vi "UpdateData.vi"(8 "error in (no error)":errorcluster, 10 "Select Conditions Criteria":T1, 11 "object in":refnum<class "TableLogger_Actor.lvclass">) -> (0 "error out":errorcluster, 2 "Data Clusters":variant[](array[variant]), 3 "object out":refnum<class "TableLogger_Actor.lvclass">)   [LabVIEW 2014, in "TableLogger_Actor.lvlib" / "TableLogger_Actor.lvclass"]
uses:
  TableLogger_Actor.lvclass
  SelectConditionCriteria.ctl
  TableLogger_SQLite_Actor/SelectConditions.ctl
  TableLogger_Actor.lvlib
panel:
  # "Connector Pane"
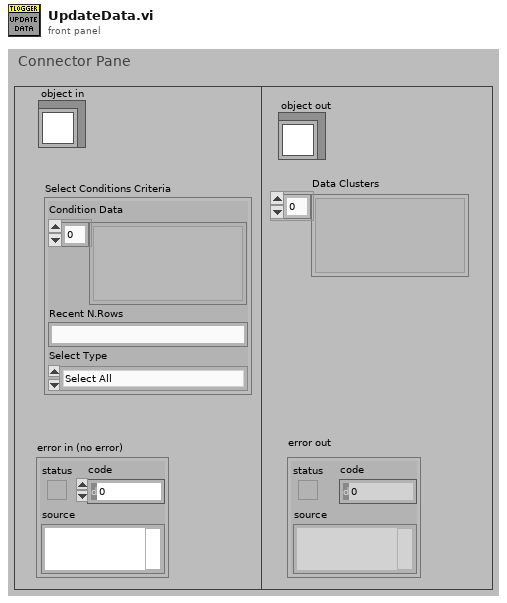
[diagram p1: front panel]
types:
  T1 = typedef "TableLogger_Actor.lvlib/SelectConditionCriteria.ctl" = cluster{"Condition Data":variant[], "Recent N.Rows":string, "Select Type":T2}
  T2 = typedef "TableLogger_Actor.lvlib/SelectConditions.ctl" = enum16{"Select All", "Select with AND Operator", "Select Most Recent Rows", "Select with OR Operator", "Select with BETWEEN Operator"}
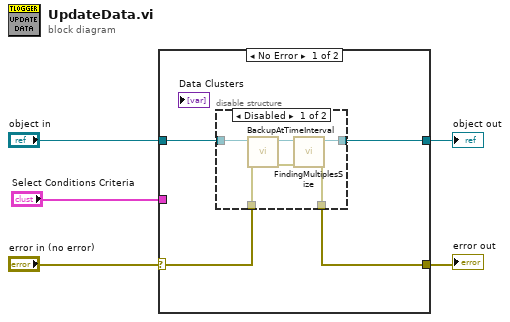
[diagram p0: block diagram]
diagram:
  n1 = case shown="No Error" "error in (no error)" {
    selector: "error in (no error)" -> [w7 w19]
    tunnel: [w8 w19] -> w4
    tunnel: [w9 w18] -> w2
    tunnel: "object in" -> [w6 w18]
    tunnel: "Select Conditions Criteria" -> [_ _]
    frame No Error {
      n2 = disable-structure shown="Disabled" {
        disable-tunnel: [w15 w17] -> w9
        disable-tunnel: [w14 w16] -> w8
        disable-tunnel: w7 -> [w13 w16]
        disable-tunnel: w6 -> [w11 w17]
        frame Disabled {
          n3 = call "BackupAtTimeInterval.vi"("error in (no error)"=w13, "object in"=w11) -> ("error out"=w12:errorcluster, "object out"=w10:refnum<class "TableLogger_Actor.lvclass">)  [unwired: 8 in]
          n4 = call "FindingMultiplesSize.vi"("error in (no error)"=w12, "TableLogger_Actor in"=w10) -> ("error out"=w14:errorcluster, "TableLogger_Actor out"=w15:refnum<class "TableLogger_Actor.lvclass">)  [unwired: 7 in, 1 out]
        }
        frame Enabled {
        }
      }
    }
    frame Error {
    }
  }
  "error out" <- w4
  "object out" <- w2
